vi "Byte Buffer.Create.vi"(8 "error in (no error)":errorcluster, 10 "byte order (big-endian)":T1(ring), 11 "size":u64) -> (0 "error out":errorcluster, 3 "Byte Buffer":refnum<class "Byte Buffer.lvclass">)   [LabVIEW 2016, in "VeriStand Data.lvlib" / "Byte Buffer.lvclass"]
doc: "Creates a new Byte Buffer instance."
uses:
  Byte Buffer.lvclass
  Byte Buffer.lvclass/Byte Buffer.ctl
  Byte Buffer.Set Buffer Pointer.vi
  Byte Buffer.Set Buffer Size.vi
  Byte Buffer.Set Buffer Length.vi
  Byte Buffer.Set Byte Order.vi
  VeriStand Data.lvlib
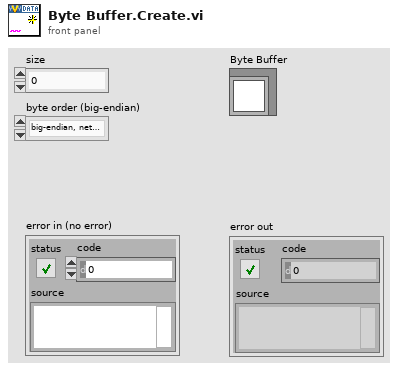
[diagram p1: front panel]
types:
  T1 = enum16{"big-endian, network order", "native, host order", "little-endian"}
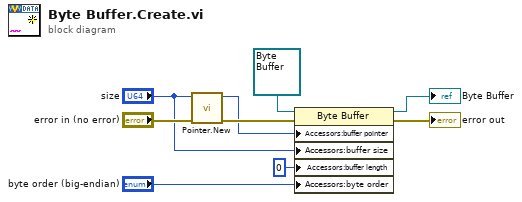
[diagram p0: block diagram]
diagram:
  n1 = call "Pointer.New.vi"("error in (no error)"="error in (no error)", "size in bytes"="size") -> ("error out"=w6:errorcluster, "pointer"=w1:u64)  [unwired: 8 in]
  n2 = property class="Byte Buffer"(reference=refnum<class "Byte Buffer.lvclass"> refnum ("VeriStand Data.lvlib:Byte Buffer"), error in=w6, "Accessors:buffer pointer"=w1, "Accessors:buffer size"="size", "Accessors:buffer length"=u64 0 ("buffer length"), "Accessors:byte order"="byte order (big-endian)") -> (reference out=→"Byte Buffer":refnum<class "Byte Buffer.lvclass">, error out=→"error out":errorcluster)
